vi "Insert all TDCHits.vi"(8 "error in (no error)":errorcluster, 10 "TDCHits":T1[](array[typedef])) -> (0 "error out":errorcluster, 1 "Nmofhits":i64[](array[numeric]), 2 "Buffer overflow out":bool)   [LabVIEW 2016]
uses:
  HPTDC Driver Library Folder/Library files/Typedefs/TDCHit.ctl
  HPTDC Driver Library Folder/HPTDC Driver Library.lvlib
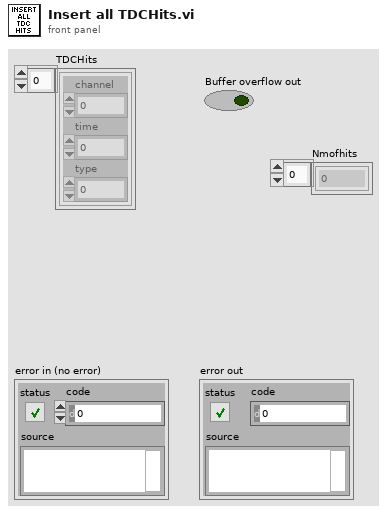
[diagram p1: front panel]
types:
  T1 = typedef "HPTDC Driver Library.lvlib/TDCHit.ctl" = cluster{"channel":u8, "time":u64, "type":u8}
  T2 = enum16{"InsertHits", "GetHits", "GetHitsDestructive"}
  T3 = enum16{"InsertHits", "GetHits", "GetHitsDestructive", "GetNumOfHits"}
  T4 = typedef "Semaphore RefNum" = refnum<k1>
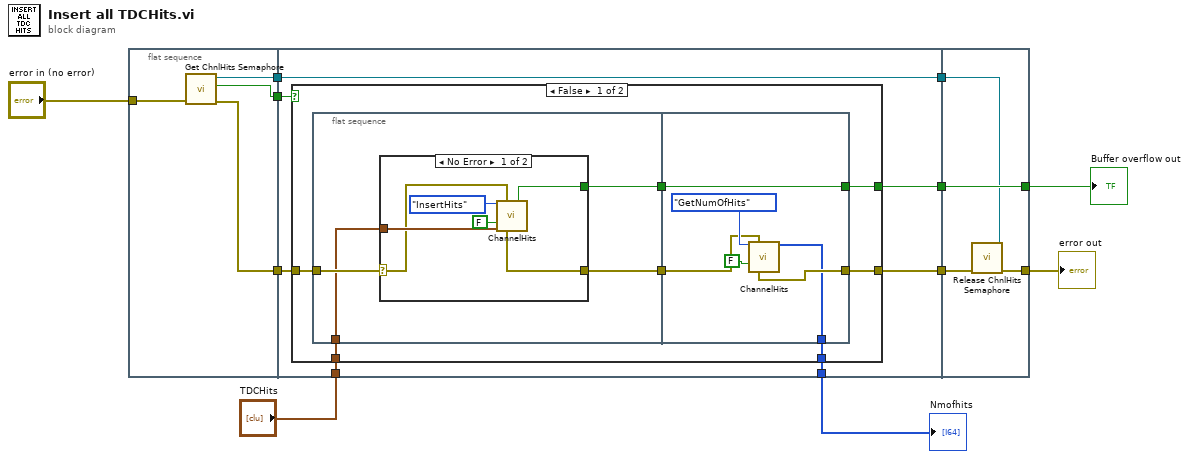
[diagram p0: block diagram]
diagram:
  n1 = flat-sequence {
    tunnel: [w15] -> w11
    tunnel: [w14] -> w6
    tunnel: [w13] -> w5
    tunnel: "error in (no error)" -> [w12]
    tunnel: w11 -> [w20]
    tunnel: "TDCHits" -> [w19]
    tunnel: [w22] -> w9
    tunnel: [w21] -> w8
    tunnel: [w18] -> w7
    tunnel: w6 -> [w18]
    tunnel: w5 -> [w17]
    tunnel: [w16] -> w2
    tunnel: [w51] -> w1
    tunnel: [w48] -> w4
    tunnel: w9 -> [w49]
    tunnel: w8 -> [w51]
    tunnel: w7 -> [w50]
    frame #0 {
      n2 = call "Get ChnlHits Semaphore.vi"("error in (no error)"=w12) -> ("error out"=w15:errorcluster, "timed out"=w13:bool, "Refnum out"=w14:T4)  [unwired: 8 in]
    }
    frame #1 {
      n3 = case shown="False" w17 {
        tunnel: [w29 w47] -> w22
        tunnel: [w28 _] -> w21
        tunnel: w20 -> [w27 w47]
        tunnel: w19 -> [w26 _]
        tunnel: [w23 _] -> w16
        frame False {
          n4 = flat-sequence {
            tunnel: w27 -> [w31]
            tunnel: w26 -> [w30]
            tunnel: [w33] -> w25
            tunnel: [w32] -> w24
            tunnel: [w46] -> w28
            tunnel: [w43] -> w29
            tunnel: w25 -> [w44]
            tunnel: w24 -> [w46]
            tunnel: [w42] -> w23
            frame #0 {
              n5 = case shown="No Error" w31 {
                selector: w31 -> [w34 w40]
                tunnel: [w38 w40] -> w33
                tunnel: w30 -> [w37 _]
                tunnel: [w36 _] -> w32
                frame No Error {
                  n6 = call "ChannelHits.vi"("Action"=T2."InsertHits", "error in"=w34, "Assert Semaphore"=FALSE, "TDCHits"=w37) -> ("Buffer overflow"=w36:bool, "Error out"=w38:errorcluster)  [unwired: 4 in, 6 out]
                }
                frame Error {
                }
              }
            }
            frame #1 {
              n7 = call "ChannelHits.vi"("Action"=T3."GetNumOfHits", "error in"=w44, "Assert Semaphore"=FALSE) -> ("Hits"=w42:u64[], "Error out"=w43:errorcluster)  [unwired: 5 in, 6 out]
            }
          }
        }
        frame True {
        }
      }
    }
    frame #2 {
      n8 = call "Release ChnlHits Semaphore.vi"("Refnum out"=w50, "error in (no error)"=w49) -> ("error out"=w48:errorcluster)  [unwired: 9 in]
    }
  }
  "Buffer overflow out" <- w1
  "error out" <- w4
  "Nmofhits" <- w2
